vi "Get Joysticks 2015.vi"() -> (0 "Robot Controls":T1)   [LabVIEW 2014]
uses:
  Robot Control Outputs 2015.ctl
  Global Variables/Refnum Names.vi
  <vilib>/Rock Robotics/WPI/Joystick/WPI_JoystickGetSetRefNum.vi
panel:
  # "CB = control board"
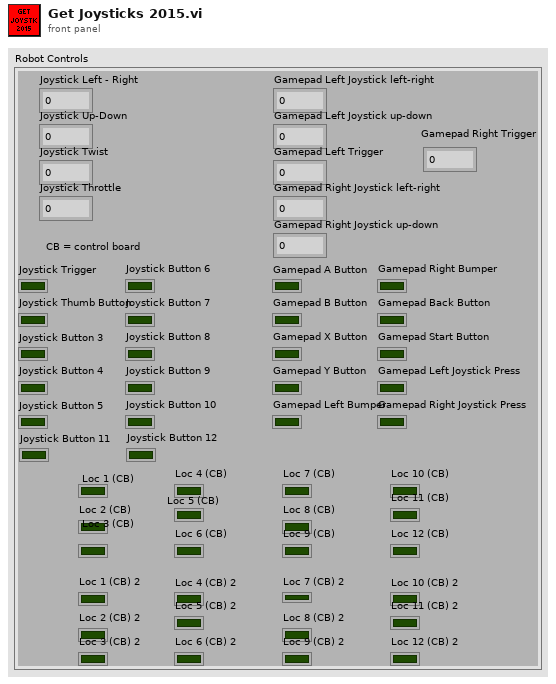
[diagram p1: front panel]
types:
  T1 = typedef "Robot Control Outputs 2015.ctl" = cluster{"Gamepad Left Joystick left-right":dbl, "Gamepad Left Joystick up-down":dbl, "Gamepad A Button":bool, "Gamepad B Button":bool, "Gamepad X Button":bool, "Gamepad Y Button":bool, "Gamepad Left Bumper":bool, "Gamepad Right Bumper":bool, "Gamepad Back Button":bool, "Gamepad Start Button":bool, "Gamepad Left Joystick Press":bool, "Gamepad Right Joystick Press":bool, "Joystick Trigger":bool, "Joystick Thumb Button":bool, "Joystick Button 3":bool, "Joystick Button 4":bool, "Joystick Button 5":bool, "Joystick Button 6":bool, "Joystick Button 7":bool, "Joystick Button 8":bool, "Joystick Button 9":bool, "Joystick Button 10":bool, "Gamepad Left Trigger":dbl, "Gamepad Right Joystick left-right":dbl, "Gamepad Right Joystick up-down":dbl, "Joystick Left - Right":dbl, "Joystick Up-Down":dbl, "Joystick Twist":dbl, "Joystick Throttle":dbl, "Loc 1 (CB)":bool, "Loc 4 (CB)":bool, "Gamepad Right Trigger":dbl, "Loc 2 (CB)":bool, "Loc 3 (CB)":bool, "Loc 5 (CB)":bool, "Loc 6 (CB)":bool, "Loc 7 (CB)":bool, "Loc 10 (CB)":bool, "Loc 8 (CB)":bool, "Loc 9 (CB)":bool, "Loc 11 (CB)":bool, "Loc 12 (CB)":bool, "Joystick Button 11":bool, "Joystick Button 12":bool, "Loc 1 (CB) 2":bool, "Loc 4 (CB) 2":bool, "Loc 2 (CB) 2":bool, "Loc 3 (CB) 2":bool, "Loc 5 (CB) 2":bool, "Loc 6 (CB) 2":bool, "Loc 7 (CB) 2":bool, "Loc 10 (CB) 2":bool, "Loc 8 (CB) 2":bool, "Loc 9 (CB) 2":bool, "Loc 11 (CB) 2":bool, "Loc 12 (CB) 2":bool}
  T2 = typedef "WPI_JoystickDevRef.ctl" = cluster{"Device":T3}
  T3 = typedef "WPI_JoystickDeviceEnum.ctl" = enum16{"USB 0", "USB 1", "USB 2", "USB 3", "USB 4", "USB 5"}
  T4 = cluster{"Axes[0]":dbl, "Axes[1]":dbl, "Axes[2]":dbl, "Axes[3]":dbl, "Axes[4]":dbl, "Axes[5]":dbl, "Axes[6]":dbl, "Axes[7]":dbl, "Axes[8]":dbl}
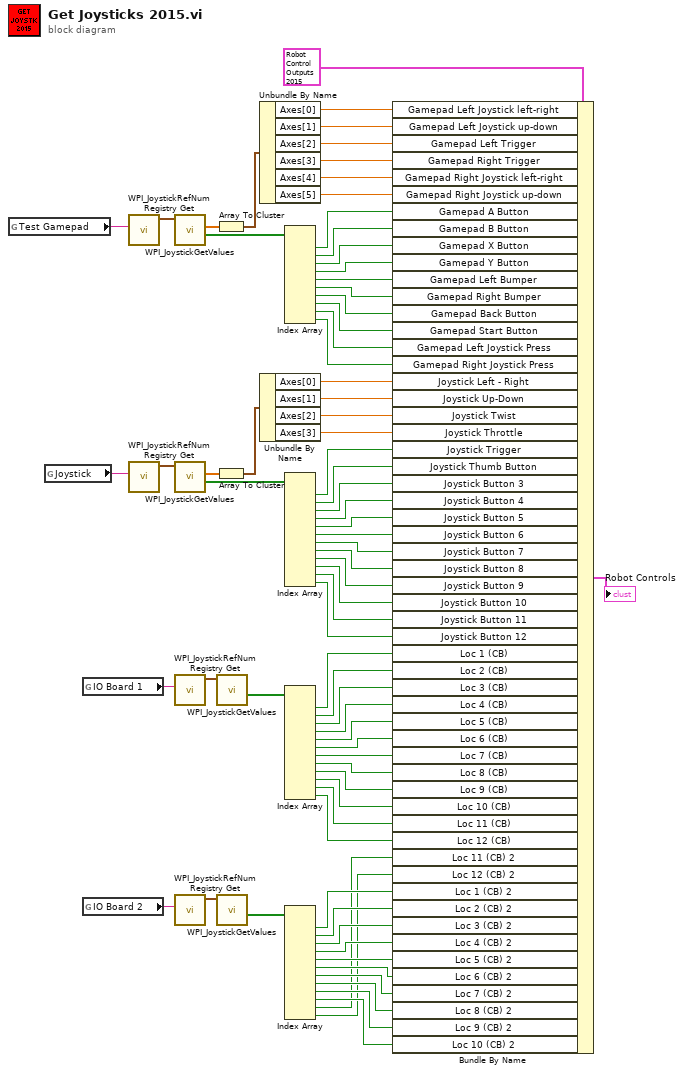
[diagram p0: block diagram]
diagram:
  n1 = global read "Refnum Names.vi" "Test Gamepad"() -> (w49:string)
  n2 = global read "Refnum Names.vi" "Joystick"() -> (w48:string)
  n3 = global read "Refnum Names.vi" "IO Board 1"() -> (w36:string)
  n4 = global read "Refnum Names.vi" "IO Board 2"() -> (w15:string)
  n5 = call <vilib>:"WPI_JoystickRefNum Registry Get.vi"("refnum name"=w49) -> ("JoystickDevRef"=w74:T2)  [unwired: 9 in, 1 out]
  n6 = call <vilib>:"WPI_JoystickRefNum Registry Get.vi"("refnum name"=w48) -> ("JoystickDevRef"=w73:T2)  [unwired: 9 in, 1 out]
  n7 = call <vilib>:"WPI_JoystickGetValues.vi"("JoystickDevRef"=w74) -> ("Buttons"=w66:bool[], "Axes"=w65:dbl[])  [unwired: 6 in, 3 out]
  n8 = call <vilib>:"WPI_JoystickGetValues.vi"("JoystickDevRef"=w73) -> ("Buttons"=w67:bool[], "Axes"=w68:dbl[])  [unwired: 6 in, 3 out]
  n9 = call <vilib>:"WPI_JoystickRefNum Registry Get.vi"("refnum name"=w36) -> ("JoystickDevRef"=w35:T2)  [unwired: 9 in, 1 out]
  n10 = call <vilib>:"WPI_JoystickRefNum Registry Get.vi"("refnum name"=w15) -> ("JoystickDevRef"=w14:T2)  [unwired: 9 in, 1 out]
  n11 = Array To Cluster(array=w65) -> (cluster=w64:T4)
  n12 = Array To Cluster(array=w68) -> (cluster=w25:T4)
  n13 = call <vilib>:"WPI_JoystickGetValues.vi"("JoystickDevRef"=w35) -> ("Buttons"=w34:bool[])  [unwired: 6 in, 4 out]
  n14 = call <vilib>:"WPI_JoystickGetValues.vi"("JoystickDevRef"=w14) -> ("Buttons"=w13:bool[])  [unwired: 6 in, 4 out]
  n15 = Unbundle By Name(w64) -> ("Axes[0]"=w72:dbl, "Axes[1]"=w71:dbl, "Axes[2]"=w47:dbl, "Axes[3]"=w70:dbl, "Axes[4]"=w69:dbl, "Axes[5]"=w46:dbl)
  n16 = Unbundle By Name(w25) -> ("Axes[0]"=w56:dbl, "Axes[1]"=w55:dbl, "Axes[2]"=w54:dbl, "Axes[3]"=w26:dbl)
  n17 = Index Array(array=w66) -> (element #1=w44:bool, element #2=w63:bool, element #3=w62:bool, element #4=w61:bool, element #5=w45:bool, element #6=w60:bool, element #7=w52:bool, element #8=w59:bool, element #9=w58:bool, element #10=w57:bool)  [unwired: 10 in]
  n18 = Index Array(array=w67) -> (element #1=w53:bool, element #2=w27:bool, element #3=w43:bool, element #4=w42:bool, element #5=w17:bool, element #6=w41:bool, element #7=w40:bool, element #8=w39:bool, element #9=w38:bool, element #10=w37:bool, element #11=w18:bool, element #12=w16:bool)  [unwired: 12 in]
  n19 = Index Array(array=w34) -> (element #1=w23:bool, element #2=w24:bool, element #3=w33:bool, element #4=w19:bool, element #5=w31:bool, element #6=w32:bool, element #7=w30:bool, element #8=w29:bool, element #9=w28:bool, element #10=w22:bool, element #11=w21:bool, element #12=w20:bool)  [unwired: 12 in]
  n20 = Index Array(array=w13) -> (element #1=w12:bool, element #2=w11:bool, element #3=w10:bool, element #4=w9:bool, element #5=w8:bool, element #6=w7:bool, element #7=w6:bool, element #8=w5:bool, element #9=w4:bool, element #10=w3:bool, element #11=w2:bool, element #12=w1:bool)  [unwired: 12 in]
  n21 = Bundle By Name(cluster=T1 {"Gamepad Left Joystick left-right"=0.0, "Gamepad Left Joystick up-down"=0.0, "Gamepad A Button"=FALSE, "Gamepad B Button"=FALSE, "Gamepad X Button"=FALSE, "Gamepad Y Button"=FALSE, "Gamepad Left Bumper"=FALSE, "Gamepad Right Bumper"=FALSE, "Gamepad Back Button"=FALSE, "Gamepad Start Button"=FALSE, "Gamepad Left Joystick Press"=FALSE, "Gamepad Right Joystick Press"=FALSE, "Joystick Trigger"=FALSE, "Joystick Thumb Button"=FALSE, "Joystick Button 3"=FALSE, "Joystick Button 4"=FALSE, "Joystick Button 5"=FALSE, "Joystick Button 6"=FALSE, "Joystick Button 7"=FALSE, "Joystick Button 8"=FALSE, "Joystick Button 9"=FALSE, "Joystick Button 10"=FALSE, "Gamepad Left Trigger"=0.0, "Gamepad Right Joystick left-right"=0.0, "Gamepad Right Joystick up-down"=0.0, "Joystick Left - Right"=0.0, "Joystick Up-Down"=0.0, "Joystick Twist"=0.0, "Joystick Throttle"=0.0, "Loc 1 (CB)"=FALSE, "Loc 4 (CB)"=FALSE, "Gamepad Right Trigger"=0.0, "Loc 2 (CB)"=FALSE, "Loc 3 (CB)"=FALSE, "Loc 5 (CB)"=FALSE, "Loc 6 (CB)"=FALSE, "Loc 7 (CB)"=FALSE, "Loc 10 (CB)"=FALSE, "Loc 8 (CB)"=FALSE, "Loc 9 (CB)"=FALSE, "Loc 11 (CB)"=FALSE, "Loc 12 (CB)"=FALSE, "Joystick Button 11"=FALSE, "Joystick Button 12"=FALSE, "Loc 1 (CB) 2"=FALSE, "Loc 4 (CB) 2"=FALSE, "Loc 2 (CB) 2"=FALSE, "Loc 3 (CB) 2"=FALSE, "Loc 5 (CB) 2"=FALSE, "Loc 6 (CB) 2"=FALSE, "Loc 7 (CB) 2"=FALSE, "Loc 10 (CB) 2"=FALSE, "Loc 8 (CB) 2"=FALSE, "Loc 9 (CB) 2"=FALSE, "Loc 11 (CB) 2"=FALSE, "Loc 12 (CB) 2"=FALSE} ("Pilot-CoPilot Gamepad Controls 2"), "Gamepad Left Joystick left-right"=w72, "Gamepad Left Joystick up-down"=w71, "Gamepad Left Trigger"=w47, "Gamepad Right Trigger"=w70, "Gamepad Right Joystick left-right"=w69, "Gamepad Right Joystick up-down"=w46, "Gamepad A Button"=w44, "Gamepad B Button"=w63, "Gamepad X Button"=w62, "Gamepad Y Button"=w61, "Gamepad Left Bumper"=w45, "Gamepad Right Bumper"=w60, "Gamepad Back Button"=w52, "Gamepad Start Button"=w59, "Gamepad Left Joystick Press"=w58, "Gamepad Right Joystick Press"=w57, "Joystick Left - Right"=w56, "Joystick Up-Down"=w55, "Joystick Twist"=w54, "Joystick Throttle"=w26, "Joystick Trigger"=w53, "Joystick Thumb Button"=w27, "Joystick Button 3"=w43, "Joystick Button 4"=w42, "Joystick Button 5"=w17, "Joystick Button 6"=w41, "Joystick Button 7"=w40, "Joystick Button 8"=w39, "Joystick Button 9"=w38, "Joystick Button 10"=w37, "Joystick Button 11"=w18, "Joystick Button 12"=w16, "Loc 1 (CB)"=w23, "Loc 2 (CB)"=w24, "Loc 3 (CB)"=w33, "Loc 4 (CB)"=w19, "Loc 5 (CB)"=w31, "Loc 6 (CB)"=w32, "Loc 7 (CB)"=w30, "Loc 8 (CB)"=w29, "Loc 9 (CB)"=w28, "Loc 10 (CB)"=w22, "Loc 11 (CB)"=w21, "Loc 12 (CB)"=w20, "Loc 11 (CB) 2"=w2, "Loc 12 (CB) 2"=w1, "Loc 1 (CB) 2"=w12, "Loc 2 (CB) 2"=w11, "Loc 3 (CB) 2"=w10, "Loc 4 (CB) 2"=w9, "Loc 5 (CB) 2"=w8, "Loc 6 (CB) 2"=w7, "Loc 7 (CB) 2"=w6, "Loc 8 (CB) 2"=w5, "Loc 9 (CB) 2"=w4, "Loc 10 (CB) 2"=w3) -> (→"Robot Controls":T1)
